vi "Write Increment Key Binding.vi"(5 "Increment Key Binding":T1, 9 "Numeric in":refnum<class "Numeric.lvclass">) -> (3 "Numeric out":refnum<class "Numeric.lvclass">)   [LabVIEW 2014, in "Numeric.lvclass"]
uses:
  Numeric.lvclass
  <vilib>/Utility/miscctls.llb/LVKeyTypeDef.ctl
  Numeric.lvclass/Numeric.ctl
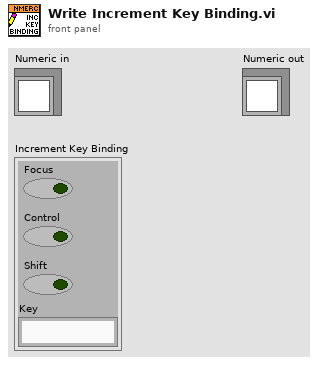
[diagram p1: front panel]
types:
  T1 = typedef "LVKeyTypeDef.ctl" = cluster{"Focus":bool, "Control":bool, "Shift":bool, "Key":string}
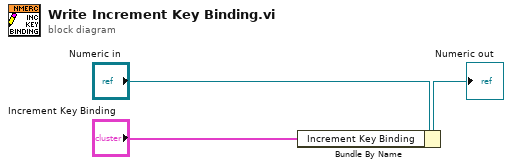
[diagram p0: block diagram]
diagram:
  n1 = Bundle By Name(cluster="Numeric in", "Increment Key Binding"="Increment Key Binding") -> (→"Numeric out":refnum<class "Numeric.lvclass">)
